vi "PressureSetpointData.vi"() -> ()   [LabVIEW 2016]
panel:
  out "Ctr Pressure":dbl=199.54651412930238
  out "Set Pressures":dbl[][](array[numeric])=[[665.1538332158755, 622.4106177021335]]
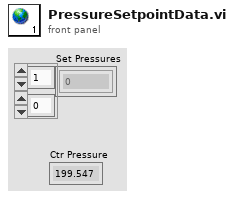
[diagram p1: front panel]
diagram:
